vi "parse-temp-string.vi"(9 "read buffer in":string=">+028.20+888888+888888+888888+888888+888888+888888", 11 "Thermocouples":T1) -> (1 "csv":string, 3 "Thermocouples":T1)   [LabVIEW 2020]
uses:
  <vilib>/regexp/Match Regular Expression.xnode
  controls/depreciated/thermocouple-data-cluster.ctl
panel:
  out "result string 3":string
  out "result string 2":string
  out "result string":string
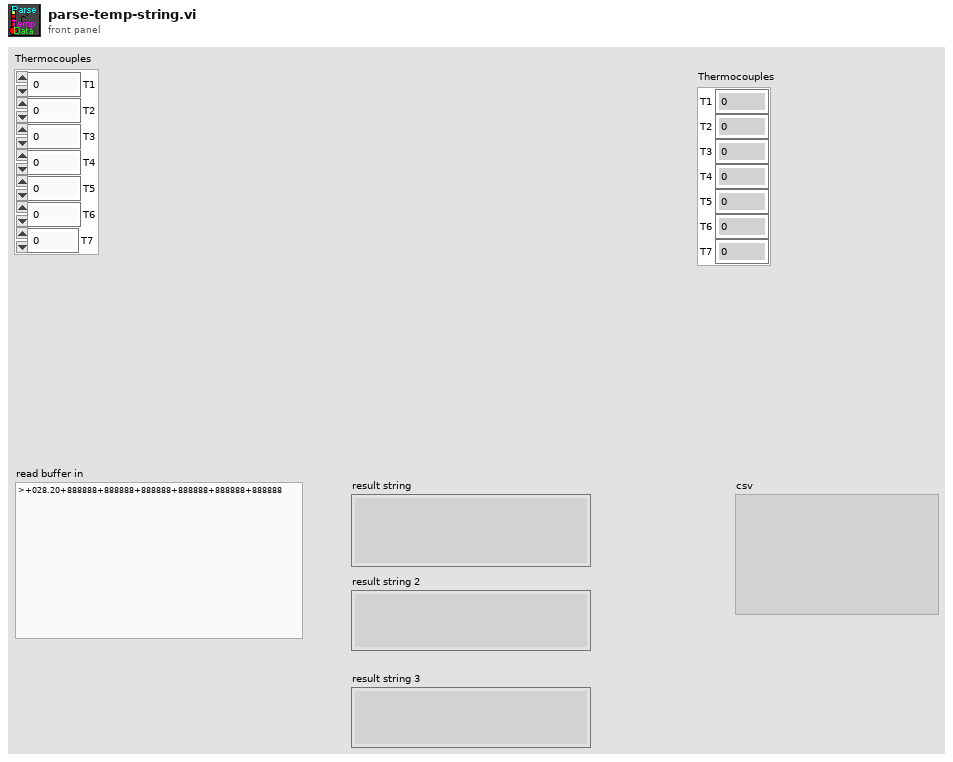
[diagram p1: front panel]
types:
  T1 = typedef "thermocouple-data-cluster.ctl" = cluster{"T1":dbl, "T2":dbl, "T3":dbl, "T4":dbl, "T5":dbl, "T6":dbl, "T7":dbl}
  T2 = cluster{"Thermocouples[0]":dbl, "Thermocouples[1]":dbl, "Thermocouples[2]":dbl, "Thermocouples[3]":dbl, "Thermocouples[4]":dbl, "Thermocouples[5]":dbl, "Thermocouples[6]":dbl, "Thermocouples[7]":dbl, "Thermocouples[8]":dbl}
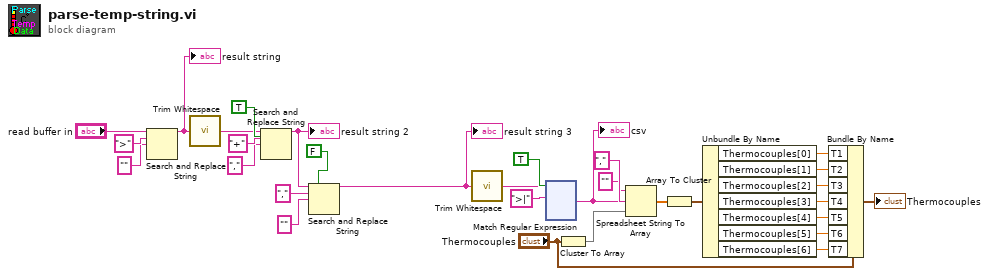
[diagram p0: block diagram]
diagram:
  n1 = Search and Replace String(input string="read buffer in", search string=">", replace string="" ("replace string (\"\")")) -> (result string=w5:string)  [unwired: 5 in, 3 out]
  "result string" <- w5
  n2 = call <vilib>:"Trim Whitespace.vi"("string"=w5) -> ("trimmed string"=w4:string)  [unwired: 1 in]
  n3 = Search and Replace String(replace all?=TRUE ("replace all? (F)"), input string=w4, search string="+", replace string="," ("replace string (\"\")")) -> (result string=w10:string)  [unwired: 4 in, 3 out]
  "result string 2" <- w10
  n4 = Search and Replace String(replace all?=FALSE ("replace all? (F)"), input string=w10, search string=",", replace string="" ("replace string (\"\")")) -> (result string=w2:string)  [unwired: 4 in, 3 out]
  "result string 3" <- w2
  n5 = call <vilib>:"Trim Whitespace.vi"("string"=w2) -> ("trimmed string"=w3:string)  [unwired: 1 in]
  n6 = xnode "Match Regular Expression"("input string"=w3, "regular expression"=">|", "multiline? (F)"=TRUE) -> ("after match"=w1:string)  [unwired: 3 in, 4 out]
  "csv" <- w1
  n7 = Cluster To Array(cluster="Thermocouples") -> (array=w27:dbl[])
  n8 = Spreadsheet String To Array(delimiter (Tab)=",", format string="", spreadsheet string=w1, array type (2D Dbl)=w27) -> (array=w28:dbl[])
  n9 = Array To Cluster(array=w28) -> (cluster=w29:T2)
  n10 = Unbundle By Name(w29) -> ("Thermocouples[0]"=w26:dbl, "Thermocouples[1]"=w24:dbl, "Thermocouples[2]"=w23:dbl, "Thermocouples[3]"=w22:dbl, "Thermocouples[4]"=w21:dbl, "Thermocouples[5]"=w20:dbl, "Thermocouples[6]"=w19:dbl)
  n11 = Bundle By Name(cluster="Thermocouples", "T1"=w26, "T2"=w24, "T3"=w23, "T4"=w22, "T5"=w21, "T6"=w20, "T7"=w19) -> (→"Thermocouples":T1)
